vi "featureXMLExpression.vi"(10 "xmlParser 0":string[](array[string]), 11 "String in":string) -> (1 "string":string, 2 "String 2":string, 3 "String":string)   [LabVIEW 2018]
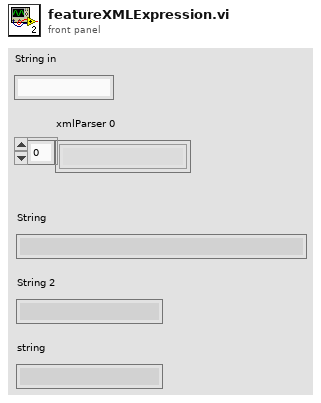
[diagram p1: front panel]
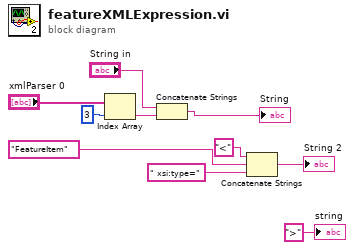
[diagram p0: block diagram]
diagram:
  n1 = Index Array(array="xmlParser 0", index=3) -> (element=w3:string)
  n2 = Concatenate Strings("String in", w3) -> (→"String":string)
  n3 = Concatenate Strings("<" ("string"), "FeatureItem", " xsi:type=") -> (→"String 2":string)
  "string" <- ">" ("string")
